vi "Construct.vi"() -> (0 "error out":errorcluster, 3 "SynchronousWriteCallback out":refnum<class "Synchronous Write Callback.lvclass">)   [LabVIEW 2020, in "Network Messenger.lvlib" / "Synchronous Write Callback.lvclass"]
uses:
  <vilib>/gpm_packages/@cs/Network-interface/Source/Network Messenger/Synchronous Write Callback/Synchronous Write Callback.lvclass
  <vilib>/gpm_packages/@cs/Network-interface/Source/Network Messenger/Synchronous Write Callback/Synchronous Write Callback.lvclass/Synchronous Write Callback.ctl
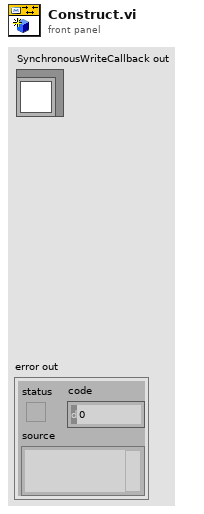
[diagram p1: front panel]
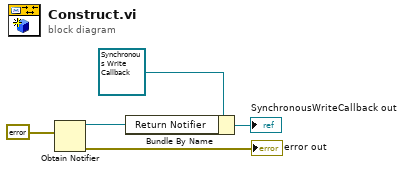
[diagram p0: block diagram]
diagram:
  n1 = Obtain Notifier(notification data type=errorcluster {"status"=FALSE, "code"=0, "source"=""} ("error in (no error)")) -> (notifier out=w3:refnum<notifier>, error out=→"error out":errorcluster)  [unwired: 3 in, 1 out]
  n2 = Bundle By Name(cluster=refnum<class "Synchronous Write Callback.lvclass"> refnum ("SynchronousWriteCallback in"), "Return Notifier"=w3) -> (→"SynchronousWriteCallback out":refnum<class "Synchronous Write Callback.lvclass">)
